vi "Sequence Sorter.vi"(2 "error in":errorcluster, 3 "sequence in":T1(array[cluster]) {"Valve" items=["None", "LOX Press", "LOX Purge", "LOX Vent", "LOX Iso", "LOX Main", "LOX Bleed", "*open*", "Fuel Press", "Fuel Purge", "Fuel Vent", "Fuel Iso", "Fuel Main", "Film Cooling", "*open*", "Ignition", "Trigger"]}) -> (0 "error out":errorcluster, 1 "sequence out":T1(array[cluster]) {"Valve" items=["None", "LOX Press", "LOX Purge", "LOX Vent", "LOX Iso", "LOX Main", "LOX Bleed", "*open*", "Fuel Press", "Fuel Purge", "Fuel Vent", "Fuel Iso", "Fuel Main", "Film Cooling", "*open*", "Ignition", "Trigger"]})   [LabVIEW 2024]
uses:
  f9d632dd-b722-4371-9ee4-7d5e9a90ae0c.vi
  ce6833b3-19ad-4906-ad44-d4b5e8c938f3.vi
  5cf53b88-c2f6-46cc-83b6-9af652960e03.vi
  165fc907-ca4c-4944-97e7-f355a83536ad.vi
  <vilib>/Comparison/Equal/Equal Functor/Equal Functor.lvclass
  <vilib>/Comparison/Less/Less Functor/Less Functor.lvclass
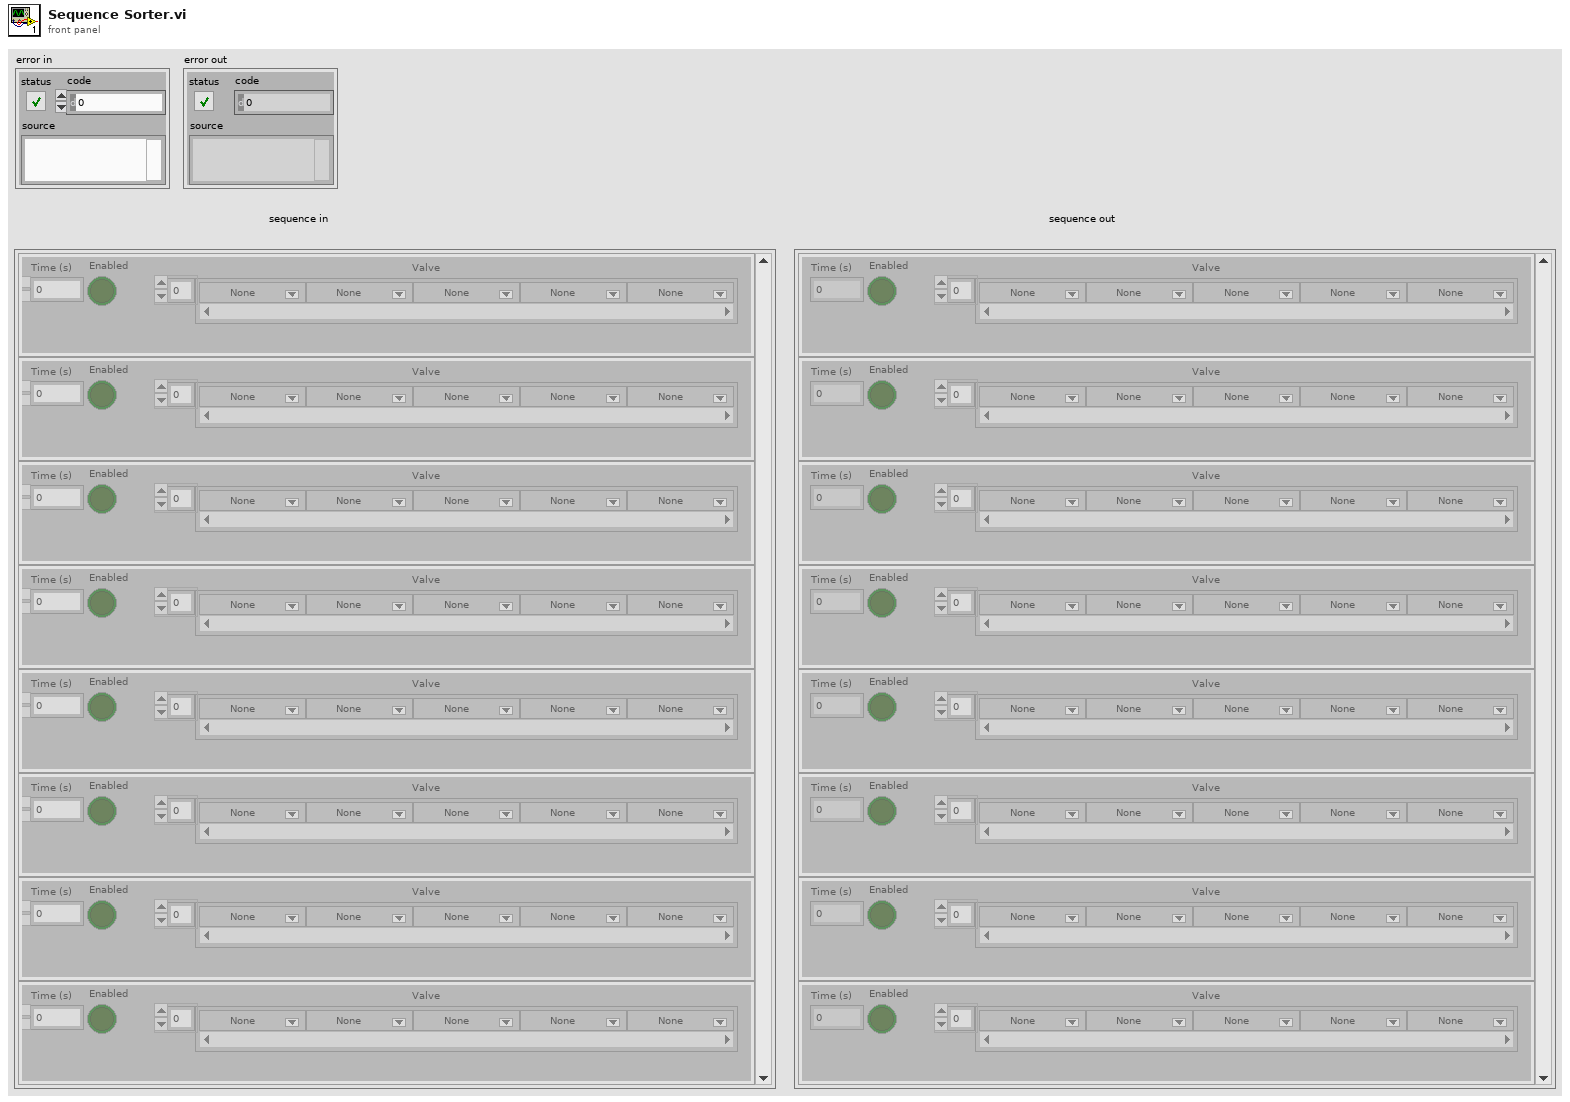
[diagram p1: front panel]
types:
  T1 = cluster{"Time (s)":dbl, "Enabled":bool, "Valve":u16[]}[]
  T2 = cluster{"Time (s)":dbl, "Enabled":bool, "Valve":u16[]}
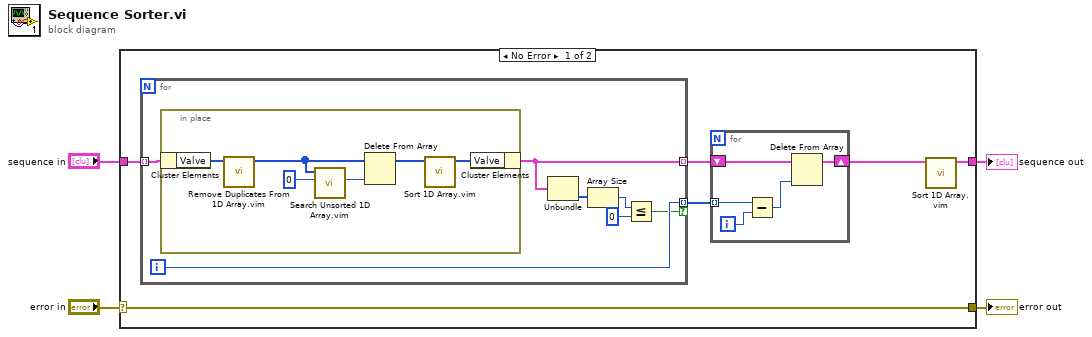
[diagram p0: block diagram]
diagram:
  n1 = case shown="No Error" "error in" {
    selector: "error in" -> [w10 w30]
    tunnel: "sequence in" -> [w9 w29]
    tunnel: [w5 w29] -> w3
    tunnel: [w10 w30] -> w1
    frame No Error {
      n2 = for {
        tunnel: w9 -> [w22] mode=indexing
        tunnel: [w21] -> w8 mode=indexing
        tunnel: [w17] -> w7 mode=indexing if=w16
        i -> [w17]
        n3 = in-place {
          n4 = in-place-cluster #1(w22) -> ("Valve"=w27:u16[])
          n5 = call "Remove Duplicates From 1D Array.vim"("array"=w27) -> ("array with duplicates removed"=w26:u16[])  [unwired: 10 in]
          n6 = call "Search Unsorted 1D Array.vim"("element"=u16 0, "unsorted 1D array"=w26) -> ("index of element"=w23:i32)  [unwired: 9 in]
          n7 = Delete From Array(array=w26, index=w23) -> (array with subset deleted=w24:u16[])  [unwired: 1 in, 1 out]
          n8 = call "Sort 1D Array.vim"("unsorted array"=w24) -> ("sorted array"=w28:u16[])  [unwired: 10 in]
          n9 = in-place-cluster #1("Valve"=w28) -> (w21:T2)
        }
        n10 = Unbundle(w21) -> ("Valve"=w20:u16[])  [unwired: 2 out]
        n11 = Array Size(array=w20) -> (size(s)=w19:i32)
        n12 = Less Or Equal?(x=w19, y=0) -> (x <= y?=w16:bool)
      }
      n13 = for {
        tunnel: w7 -> [w13] mode=indexing
        shift-right: [w14] -> w6
        shift-left: w8 -> [w15]
        i -> [w11]
        n14 = Subtract(x=w13, y=w11) -> (x-y=w12:i32)
        n15 = Delete From Array(array=w15, index=w12) -> (array with subset deleted=w14:T1)  [unwired: 1 in, 1 out]
      }
      n16 = call "Sort 1D Array.vim"("unsorted array"=w6) -> ("sorted array"=w5:T1)  [unwired: 10 in]
    }
    frame Error {
    }
  }
  "error out" <- w1
  "sequence out" <- w3
